vi "TestInitializeLocalLog_InjectMultipleEditTimeAbsRunTimeConcrete_LogEventCaptured.vi"(8 "error in (no error)":errorcluster, 11 "TestCase in":refnum<class "TestMalleableInterface.lvclass">) -> (0 "error out":errorcluster, 3 "TestCase out":refnum<class "TestMalleableInterface.lvclass">)   [LabVIEW 2017, in "TestMalleableInterface.lvclass"]
uses:
  TestMalleableInterface.lvclass
  Source/Composed Log/Log Sink/Log Sink.lvclass
  Source/LVQueue Sink/LVQueue Sink.lvclass/LVQueue Sink.ctl
  Source/Composed Log/LoggerReference/LoggerReference.lvclass/LoggerReference.ctl
  8d299841-f253-422a-a7a1-59edf70c310f.vi
  Source/Composed Log/LoggerReference/Return Aggregate Queues.vi
  Source/Composed Log/LoggerReference/Add Aggregate Log.vi
  8d299841-f253-422a-a7a1-59edf70c310f.vi/713dfd60-5520-4f5d-9a7b-9fe4433646fb.vi
  Source/Composed Log/LoggerReference/Log.vi
  Source/Composed Log/LoggerReference/Send Add Sink.vi
  Source/Composed Log/LoggerReference/Remove Stale Logs.vi
  Source/LVQueue Sink/LVQueue Sink.lvclass
  C:/CS/Internal/LabVIEW/Logger/Source/Composed Log/Log Sink/Log Sink.lvclass
  Source/Composed Log/Application Logger/Launch Worker Loop.vi
  Source/Composed Log/LoggerReference/Initialize Logger Instance.vi
  Source/Composed Log/LoggerReference/LoggerReference.lvclass
  Source/Composed Log/IErrorFormat/IErrorFormat.lvclass
  <vilib>/addons/_JKI Toolkits/VI Tester/TestCase.llb/TestCase.lvclass
  C:/Program Files (x86)/National Instruments/LabVIEW 2017/vi.lib/addons/_JKI Toolkits/VI Tester/TestCase.llb/TestCase.lvclass
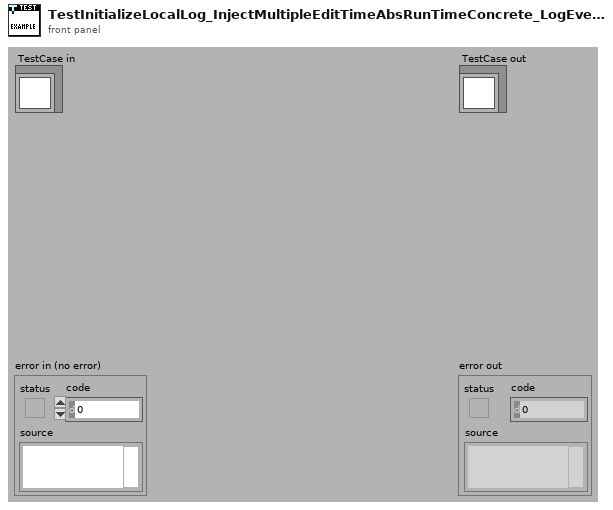
[diagram p1: front panel]
types:
  T1 = typedef "Composed Log.lvlib/Log Packet.ctl" = cluster{"Data To Log":string, "Source":string, "Event Level":T2, "Event Time":timestamp}
  T2 = typedef "Composed Log.lvlib/Log Level.ctl" = enum16{"Debug", "Info", "Warning", "Error", "Critical"}
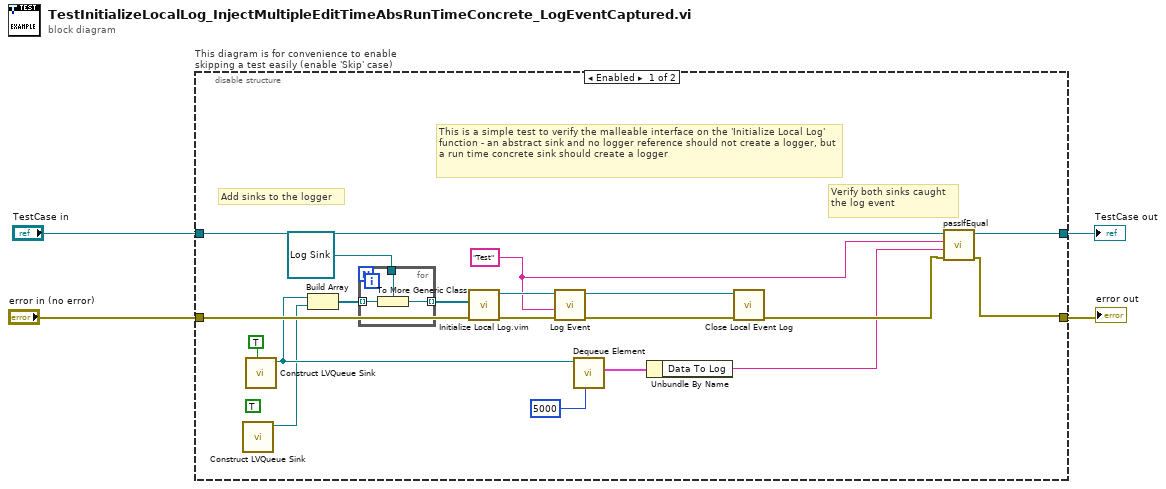
[diagram p0: block diagram]
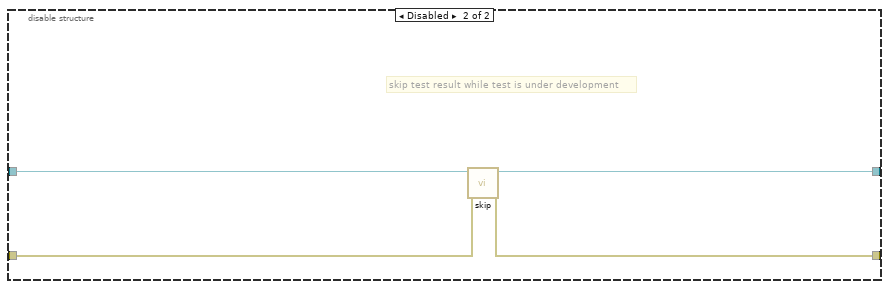
[diagram p2: hidden frame]
diagram:
  n1 = disable-structure "This diagram is for convenience to enable skipping a test easily (enable 'Skip' case)" shown="Enabled" {
    disable-tunnel: "TestCase in" -> [w14 w30]
    disable-tunnel: [w13 w28] -> w1
    disable-tunnel: [w15 w29] -> w3
    disable-tunnel: "error in (no error)" -> [w10 w27]
    frame Enabled {
      (unwired) TRUE ("User Shutdown? (F)")
      w11 = "Test" ("SourceID")
      # "This is a simple test to verify the malleable interface on the 'Initialize Local Log' function - an abstract sink and no logger reference should not create a logger, but a run time concrete sink should create a logger"
      # "Verify both sinks caught the log event"
      # "Add sinks to the logger"
      n2 = call "Construct LVQueue Sink.vi"() -> ("LVQueue Sink out"=w6:refnum<class "LVQueue Sink.lvclass">)  [unwired: 10 in, 1 out]
      n3 = call "Construct LVQueue Sink.vi"("User Shutdown? (F)"=TRUE) -> ("LVQueue Sink out"=w7:refnum<class "LVQueue Sink.lvclass">)  [unwired: 9 in, 1 out]
      n4 = Build Array(w7, w6) -> (w5:refnum<class "LVQueue Sink.lvclass">[])
      n5 = for {
        tunnel: refnum<class "Log Sink.lvclass"> refnum ("Startup Sink(s)") -> [w26]
        tunnel: [w24] -> w9 mode=indexing
        tunnel: w5 -> [w25] mode=indexing
        n6 = To More Generic Class(target class=w26, reference=w25) -> (generic class reference=w24:refnum<class "Log Sink.lvclass">)
      }
      n7 = call "Initialize Local Log.vim"("error in (no error)"=w10, "Startup Sink(s)"=w9) -> ("error out"=w19:errorcluster, "Log Instance Reference"=w20:refnum<class "LoggerReference.lvclass">)  [unwired: 7 in, 1 out]
      n8 = call "Log Event.vi"("error in (no error)"=w19, "Data To Log"=w11, "Log Instance"=w20) -> ("error out"=w22:errorcluster, "Log Instance Out"=w21:refnum<class "LoggerReference.lvclass">)  [unwired: 7 in]
      n9 = call "Dequeue Element.vi"("timeout in ms (-1)"=5000, "LVQueue Sink in"=w7) -> ("Log Packet"=w18:T1)  [unwired: 6 in, 3 out]
      n10 = Unbundle By Name(w18) -> ("Data To Log"=w12:string)
      n11 = call "Close Local Event Log.vi"("error in (no error)"=w22, "Log Instance"=w21) -> ("error out"=w16:errorcluster)  [unwired: 9 in]
      n12 = call-dynamic "passIfEqual.vi"("error in (no error)"=w16, "y"=w12, "x"=w11, "TestCase in"=w14) -> ("error out"=w15:errorcluster, "TestCase out"=w13:refnum<class "TestMalleableInterface.lvclass">)  [unwired: 6 in]
    }
    frame Disabled {
      # "skip test result while test is under development"
      n13 = call <vilib>:"skip.vi"("error in (no error)"=w27, "TestCase in"=w30) -> ("error out"=w29:errorcluster, "TestCase out"=w28:refnum<class "TestMalleableInterface.lvclass">)  [unwired: 8 in]
    }
  }
  "error out" <- w3
  "TestCase out" <- w1
